vi "Launcher.vi"() -> ()   [LabVIEW 2020]
uses:
  Abstract/Serial Device/Combo Box Devices.ctl
  UI Actor.lvclass
  C:/Program Files (x86)/National Instruments/LabVIEW 2020/vi.lib/ActorFramework/Actor/Actor.lvclass
  Implementation/Simulado/Simulado.lvclass
  D:/Users/salaz/GitHub/Puerto-COM_labview-Actor-Framework/Abstract/Serial Device/Serial Device.lvclass
  Implementation/NXP/NXP.lvclass
  Implementation/Cypress/Cypress.lvclass
  UI Actor.lvclass/UI Actor.ctl
  Write Serial Device.lvclass.vi
  <vilib>/ActorFramework/Actor/Actor.lvclass
panel:
  in  "Serial Devide Brand":T1
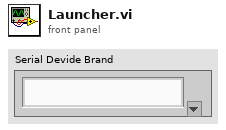
[diagram p1: front panel]
types:
  T1 = typedef "Combo Box Devices.ctl" = string
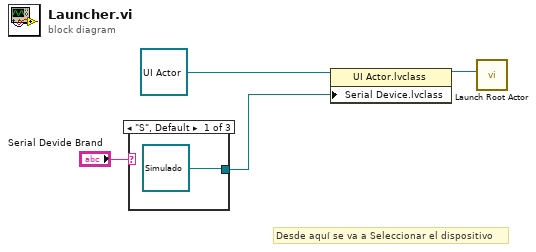
[diagram p0: block diagram]
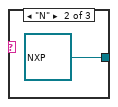
[diagram p2: hidden frame]
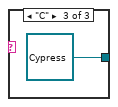
[diagram p3: hidden frame]
diagram:
  # "Desde aquí se va a Seleccionar el dispositivo"
  n1 = case shown="\"S\", Default" "Serial Devide Brand" {
    tunnel: [refnum<class "Simulado.lvclass"> refnum ("Simulado.lvclass") refnum<class "NXP.lvclass"> refnum ("NXP.lvclass") refnum<class "Cypress.lvclass"> refnum ("Cypress.lvclass")] -> w1
    frame "S", Default {
    }
    frame "N" {
    }
    frame "C" {
    }
  }
  n2 = property class="UI Actor.lvclass"(reference=refnum<class "UI Actor.lvclass"> refnum ("UI Actor.lvlib:UI Actor.lvclass"), "Serial Device.lvclass"=w1) -> (reference out=w3:refnum<class "UI Actor.lvclass">)  [unwired: 1 in, 1 out]
  n3 = call <vilib>:"Launch Root Actor.vi"("Actor"=w3) -> ()  [unwired: 9 in, 2 out]
